vi "DHE_DO_IMREAD_CONT.vi"(8 "error in":errorcluster) -> (0 "error out":errorcluster, 2 "response":string="END READ CONT")   [LabVIEW 2016]
uses:
  Common/public/vis/CMN_FVAR_action.ctl
  SDSU_GBLVariables.vi
  DBSHAND/private/vis/DatabaseHand_Element_Get(I32).vi
  DBSHAND/private/vis/DatabaseHand_Element_Get(double).vi
  DBSHAND/private/vis/DatabaseHand_Element_Set(bool).vi
  c/lib/libarcDHE.so
panel:
  out "remaining elements":string[](array[string])
  out "read prog":i32
  in  "stop":bool
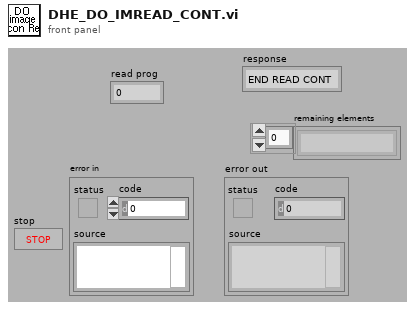
[diagram p1: front panel]
types:
  T1 = typedef "DatabaseHand_RefNum.ctl" = refnum<vi>
  T2 = typedef "CMN_FVAR_action.ctl" = enum16{"read", "write"}
  T3 = enum16{"Idle", "Exposing", "Paused", "AbortExp", "Reading", "AbortRead", "FinishedReading", "Resetting", "Reducing"}
  T4 = typedef "CMN_Buffers.ctl" = cluster{"TotalPixels":u32, "Total image bytes":u32, "Total Phys Buffers":u32, "virtual buf pixels":u32, "virtual bytes size":u32, "Remaining piece":u32, "Transfer_Buf_size":u32}
  T5 = typedef "CMN_ContStatus.ctl" = cluster{"Response":string, "power":bool, "shutter":bool, "artifdata":bool, "idlemode":bool, "reset":bool, "gain":u8, "speed":u8, "resetPCI":bool, "autoshutter":bool, "TempSetPoint":i32, "multipleextensions":bool, "displayImage":bool, "coadding":bool, "images being coadded":i32, "Operation Mode":enum16{"normal", "coadd", "fawler"}, "frames to write":cluster{"subs":bool, "reset":bool, "exposed":bool}, "fawler samples":i32, "write auto":bool, "datatype":string, "frames to display":cluster{"subs":bool, "reset":bool, "exposed":bool}, "sur":i32, "autoclear":bool}
  T6 = enum16{"Idle", "Exposing", "Paused", "AbortExp", "Reading", "AbortRead", "FinishedReading", "Resetting", "Reducing", "Initializing"}
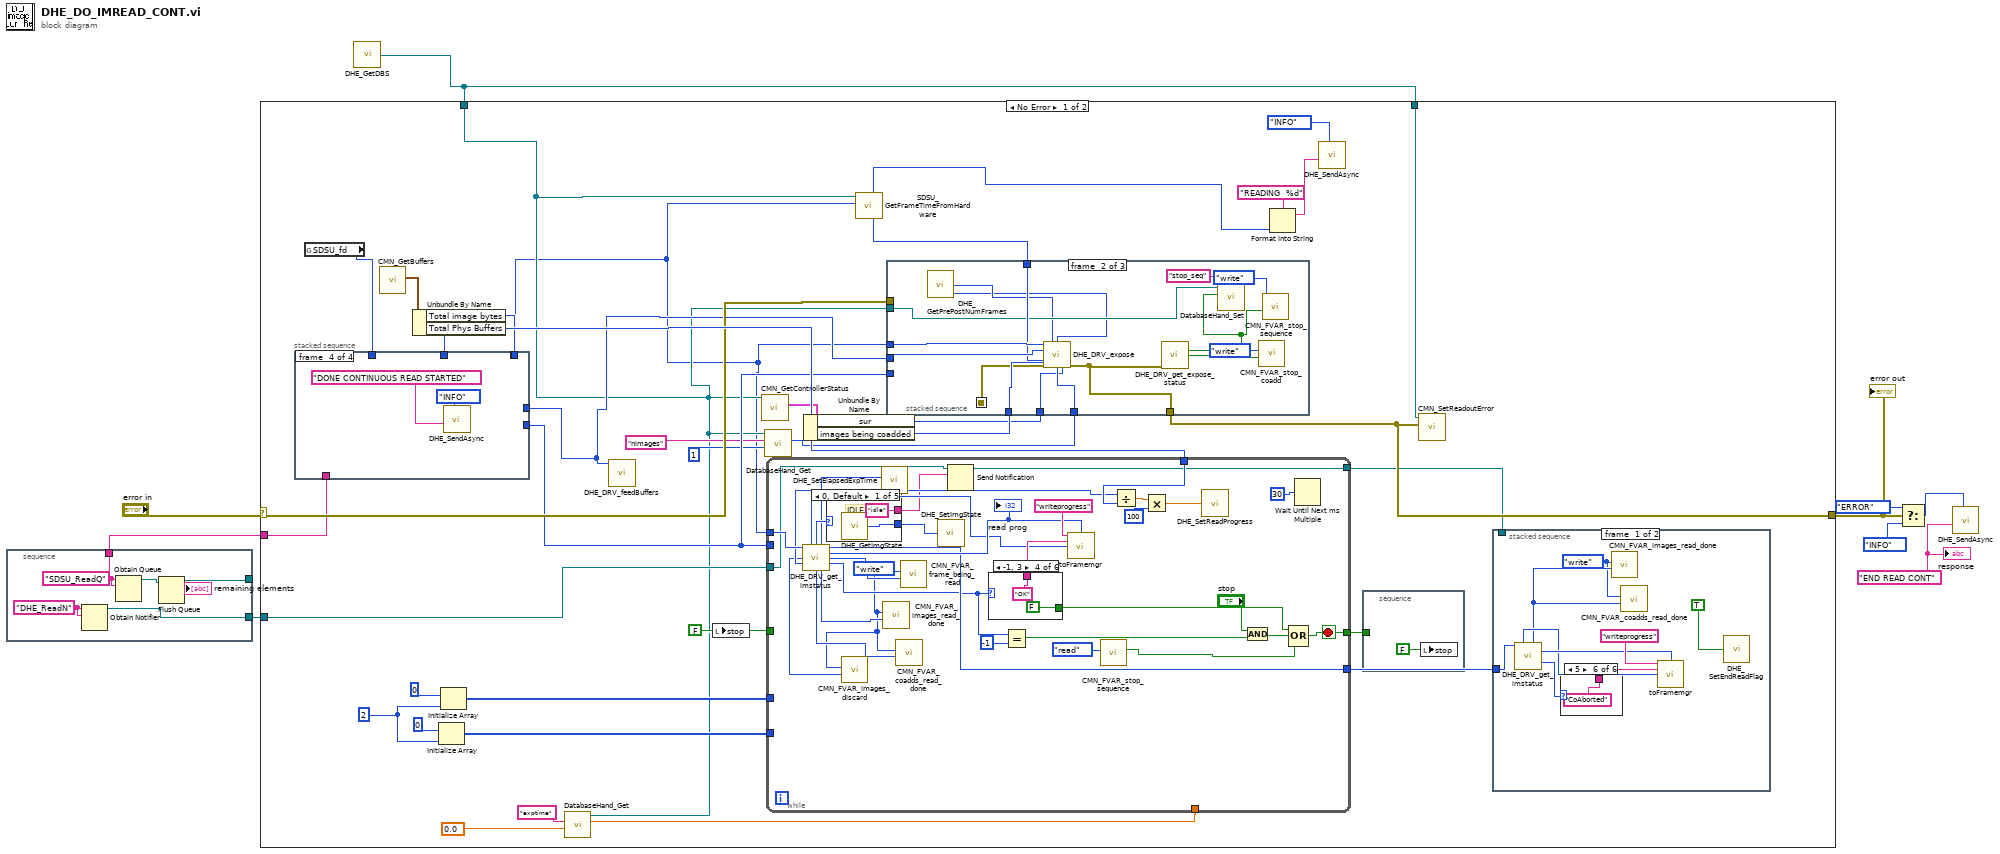
[diagram p0: block diagram]
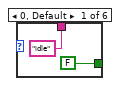
[diagram p2: hidden frame]
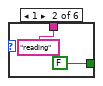
[diagram p3: hidden frame]
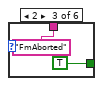
[diagram p4: hidden frame]
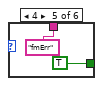
[diagram p5: hidden frame]
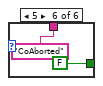
[diagram p6: hidden frame]
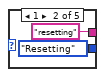
[diagram p7: hidden frame]
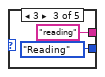
[diagram p8: hidden frame]
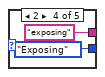
[diagram p9: hidden frame]
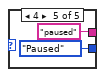
[diagram p10: hidden frame]
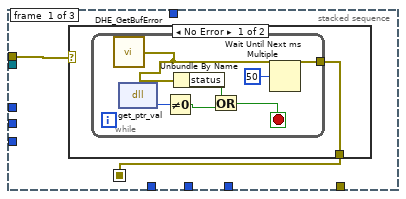
[diagram p11: hidden frame]
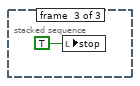
[diagram p13: hidden frame]
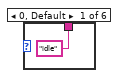
[diagram p14: hidden frame]
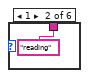
[diagram p15: hidden frame]
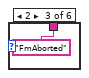
[diagram p16: hidden frame]
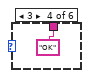
[diagram p17: hidden frame]
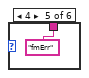
[diagram p18: hidden frame]
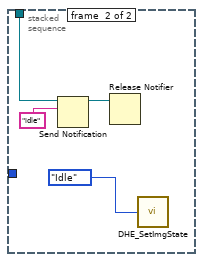
[diagram p19: hidden frame]
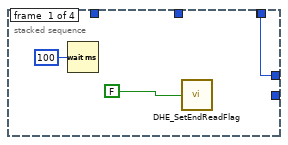
[diagram p20: hidden frame]
diagram:
  w1 = "END READ CONT" ("Message")
  n1 = stacked-sequence {
    tunnel: [w15] -> w8
    tunnel: [w13] -> _
    tunnel: [w10] -> w7
    frame #0 {
      w11 = "DHE_ReadN" ("name (unnamed)")
      w15 = "SDSU_ReadQ" ("name (unnamed)")
      n2 = Obtain Notifier(name (unnamed)=w11, notification data type=w11) -> (notifier out=w10:refnum<notifier>)  [unwired: 2 in, 2 out]
      n3 = Obtain Queue(name (unnamed)=w15, element data type=w15) -> (queue out=w14:refnum<queue>)  [unwired: 3 in, 2 out]
      n4 = Flush Queue(queue=w14) -> (queue out=w13:refnum<queue>, remaining elements=→"remaining elements":string[])  [unwired: 1 in, 1 out]
    }
  }
  n5 = call "DHE_GetDBS.vi"() -> ("DHE_DBSRef"=w6:T1)  [unwired: 9 out]
  n6 = case shown="No Error" "error in" {
    selector: "error in" -> [w43 w169]
    tunnel: [w40 w169] -> w5
    tunnel: w6 -> [w39 _]
    tunnel: w6 -> [w18 _]
    tunnel: w8 -> [w33 _]
    tunnel: w7 -> [w29 _]
    frame No Error {
      w21 = 2 ("dimension size")
      w42 = FALSE ("stop")
      n7 = global read "SDSU_GBLVariables.vi" "SDSU_fd"() -> (w17:i32)
      n8 = call "CMN_GetBuffers.vi"() -> ("BuffersDimensions"=w34:T4)  [unwired: 2 in, 9 out]
      n9 = Unbundle By Name(w34) -> ("Total image bytes"=w31:u32, "Total Phys Buffers"=w51:u32)
      n10 = stacked-sequence {
        tunnel: [_ w157 _ _] -> w41
        tunnel: w51 -> [_ w159 _ _]
        tunnel: w17 -> [_ w158 _ _]
        tunnel: w33 -> [_ _ w161 _]
        tunnel: [w154 _ _ _] -> w30
        tunnel: w31 -> [w154 _ _ _]
        tunnel: [_ w156 _ _] -> w16
        frame #0 {
          n11 = Wait (ms)(milliseconds to wait=u32 100) -> ()  [unwired: 1 out]
          n12 = call "DHE_SetEndReadFlag.vi"("DHE_read_ended"=FALSE ("readout ended")) -> ()  [unwired: 9 out]
        }
        frame #1 {
          n13 = dll-call lib="home/simager/panview/PAN/Modules/SDSU/private/c/lib/libarcDHE.so" fn="clear_exp_vals"() -> ()  [unwired: 3 in, 3 out]
          n14 = call "DHE_DRV_clear_progress_buf.vi"("fd"=w158) -> ("fd"=w156:i32)  [unwired: 1 in, 13 out]
          n15 = dll-call lib="home/simager/panview/PAN/Modules/SDSU/private/c/lib/libarcDHE.so" fn="clear_counters"() -> ()  [unwired: 3 in, 3 out]
          n16 = dll-call lib="home/simager/panview/PAN/Modules/SDSU/private/c/lib/libarcDHE.so" fn="set_bufs_per_frame" label="bufs_per_frame"("total_bufs"=w159) -> ("total_bufs"=w157:i32)  [unwired: 3 in, 3 out]
          n17 = dll-call lib="home/simager/panview/PAN/Modules/SDSU/private/c/lib/libarcDHE.so" fn="clear_discards"() -> ()  [unwired: 3 in, 3 out]
        }
        frame #2 {
          n18 = dll-call lib="home/simager/panview/PAN/Modules/SDSU/private/c/lib/libarcDHE.so" fn="set_status_expo"() -> ()  [unwired: 3 in, 3 out]
          n19 = Concatenate Strings("reading" ("command"), " " ("string"), w161) -> (w160:string)
          n20 = call "CMN_toLogical.vi"("command"=w160) -> ()  [unwired: 10 out]
        }
        frame #3 {
          n21 = call "DHE_SendAsync.vi"("type"=enum16{"ERROR", "WARNING", "INFO", "CHANGED"}."INFO", "Message"="DONE CONTINUOUS READ STARTED") -> ()  [unwired: 10 out]
        }
      }
      n22 = Initialize Array(i16 0, w21) -> (w49:i16[])
      n23 = Initialize Array(0, w21) -> (w50:i32[])
      n24 = call-poly "DatabaseHand_Get.vi"("default value"=0.0, "name"="exptime", "Database RefNum in"=w18) -> ("value"=w32:dbl)  [unwired: 2 in, 6 out]
      n25 = call "DHE_DRV_feedBuffers.vi"("bufsize"=w30) -> ()  [unwired: 10 out]
      n26 = local write "stop"(w42) -> ()
      n27 = call "CMN_GetControllerStatus.vi"("DBS Ref"=w18) -> ("ControllerStatus"=w38:T5)  [unwired: 10 out]
      n28 = call-poly "DatabaseHand_Get.vi"("default value"=1, "name"="nimages", "Database RefNum in"=w18) -> ("value"=w22:i32)  [unwired: 2 in, 6 out]
      n29 = while {
        tunnel: w49 -> [_]
        tunnel: w50 -> [_]
        tunnel: [w73] -> w44
        tunnel: [w70] -> w46
        tunnel: w51 -> [w77]
        tunnel: w16 -> [w79]
        tunnel: w42 -> [_]
        tunnel: w41 -> [_]
        tunnel: w32 -> [_]
        tunnel: w29 -> [w64]
        tunnel: [w63] -> w28
        stop <- w70 stop-if-true
        w55 = CMN_FVAR_action."write" ("action")
        n30 = call "DHE_DRV_get_imstatus.vi"("fd"=w79) -> ("ptr to buffer"=w74:u64, "image status"=w78:i16, "exposure progress"=w60:i32, "fd"=w73:i32, "buff read"=w75:i32, "fowlers_discarded"=w56:i32, "frames read"=w59:i32, "actual_buf_reads"=w72:i32, "frame status"=w68:i32, "coadds done"=w57:i32, "images done"=w58:i32)  [unwired: 1 in, 3 out]
        "read prog" <- w75
        n31 = case shown="0, Default" w78 {
          tunnel: [w96 T3."Resetting" ("ImgState") T3."Reading" ("ImgState") T3."Exposing" ("ImgState") T3."Paused" ("ImgState")] -> w61
          tunnel: ["idle" "resetting" "reading" "exposing" "paused"] -> w62
          frame 0, Default {
            # "IDLE"
            n32 = call "DHE_GetImgState.vi"() -> ("DHE_ImgState"=w96:T6)  [unwired: 9 out]
          }
          frame 1 {
          }
          frame 3 {
          }
          frame 2 {
          }
          frame 4 {
          }
        }
        n33 = call "CMN_FVAR_images_discard.vi"("value in"=w56, "action"=w55) -> ()  [unwired: 9 out]
        n34 = call "DHE_SetElapsedExpTime.vi"("ElapsedExpTime"=w60) -> ()  [unwired: 11 out]
        n35 = call "CMN_FVAR_images_read_done.vi"("value in"=w58, "action"=w55) -> ()  [unwired: 9 out]
        n36 = call "CMN_FVAR_coadds_read_done.vi"("value in"=w57, "action"=w55) -> ()  [unwired: 9 out]
        n37 = call "CMN_FVAR_frame_being_read.vi"("value in"=w59, "action"=w55) -> ()  [unwired: 9 out]
        n38 = call "DHE_SetImgState.vi"("DHE_ImgState"=w61) -> ()  [unwired: 9 out]
        n39 = Send Notification(notification=w62, notifier=w64) -> (notifier out=w63:refnum<notifier>)  [unwired: 1 in, 1 out]
        n40 = case shown="-1, 3" w68 {
          tunnel: ["idle" "reading" "FmAborted" "OK" "fmErr" "CoAborted"] -> w76
          tunnel: [FALSE FALSE TRUE FALSE TRUE FALSE] -> w65
          frame 0, Default {
          }
          frame 1 {
          }
          frame 2 {
          }
          frame -1, 3 {
          }
          frame 4 {
          }
          frame 5 {
          }
        }
        n41 = Equal?(x=w68, y=-1) -> (x = y?=w66:bool)
        n42 = call "toFramemgr.vi"("command"="writeprogress", "progress"=w75, "arg"=w76, "bufpointer"=w74) -> ()  [unwired: 5 in, 7 out]
        n43 = call "CMN_FVAR_stop_sequence.vi"("action"=CMN_FVAR_action."read") -> ("value out"=w52:bool)  [unwired: 1 in, 8 out]
        n44 = Divide(x=w72, y=w77) -> (x/y=w81:dbl)
        n45 = Multiply(x=w81, y=100) -> (x*y=w54:dbl)
        n46 = call "DHE_SetReadProgress.vi"("ReadProgress"=w54) -> ()  [unwired: 11 out]
        n47 = And(x="stop", y=w66) -> (x .and. y?=w69:bool)
        n48 = Compound Arithmetic op=OR(w65, w69, w52) -> (w70:bool)
        n49 = Wait Until Next ms Multiple(millisecond multiple=u32 30) -> ()  [unwired: 1 out]
      }
      n50 = Unbundle By Name(w38) -> ("sur"=w37:i32, "images being coadded"=w45:i32)
      n51 = call "SDSU_GetFrameTimeFromHardware.vi"("fd"=w16, "Database Ref"=w18) -> ("idle time"=w20:u32, "total exp time"=w19:u32)  [unwired: 1 in, 7 out]
      n52 = stacked-sequence {
        seq-local: [w108 _ _] -> [_ w128 _]
        tunnel: w30 -> [_ w131 _]
        tunnel: w16 -> [_ w132 _]
        tunnel: [_ w126 _] -> w40
        tunnel: w43 -> [w107 _ _]
        tunnel: w22 -> [_ w130 _]
        tunnel: w45 -> [_ w129 _]
        tunnel: w20 -> [_ w127 _]
        tunnel: w41 -> [_ _ _]
        tunnel: w37 -> [_ w125 _]
        tunnel: w18 -> [_ w124 _]
        frame #0 {
          n53 = case shown="No Error" w107 {
            selector: w107 -> [_ w116]
            tunnel: [w109 w116] -> w108
            frame No Error {
              n54 = while {
                tunnel: [w110] -> w109
                stop <- w112 stop-if-true
                n55 = call "DHE_GetBufError.vi"() -> ("DHE_BufError"=w110:errorcluster)  [unwired: 9 out]
                n56 = dll-call lib="home/simager/panview/PAN/Modules/SDSU/private/c/lib/libarcDHE.so" fn="get_ptr_val"() -> (w115:u32)  [unwired: 3 in, 2 out]
                n57 = Not Equal To 0?(x=w115) -> (x != 0?=w114:bool)
                n58 = Unbundle By Name(w110) -> ("status"=w111:bool)
                n59 = Or(x=w111, y=w114) -> (x .or. y?=w112:bool)
                n60 = Wait Until Next ms Multiple(millisecond multiple=u32 50) -> ()  [unwired: 1 out]
              }
            }
            frame Error {
            }
          }
        }
        frame #1 {
          n61 = call "DHE_GetPrePostNumFrames.vi"() -> ("DHE_PreExpose"=w122:i32, "DHE_PostExpose"=w121:i32)  [unwired: 8 out]
          n62 = call "DHE_DRV_expose.vi"("fd"=w132, "num_prevex"=w122, "num_postex"=w121, "bytes_to_receive"=w131, "expt_time"=w127, "error in (no error)"=w128, "num_coadds"=w129, "npics"=w130, "num_sur"=w125) -> ("error out"=w126:errorcluster)  [unwired: 1 in, 5 out]
          n63 = call "DHE_DRV_get_expose_status.vi"("error in (no error)"=w126) -> ("sequence stoped"=w120:bool, "coadd stoped"=w118:bool)  [unwired: 13 out]
          n64 = call-poly "DatabaseHand_Set.vi"("name"="stop_seq", "value"=w120, "Database RefNum in"=w124) -> ()  [unwired: 5 in, 4 out]
          n65 = call "CMN_FVAR_stop_coadd.vi"("value in"=w118, "action"=CMN_FVAR_action."write") -> ()  [unwired: 9 out]
          n66 = call "CMN_FVAR_stop_sequence.vi"("value in"=w120, "action"=CMN_FVAR_action."write") -> ()  [unwired: 9 out]
        }
        frame #2 {
          n67 = local write "stop"(TRUE ("stop")) -> ()
        }
      }
      n68 = Format Into String(format string="READING  %d", w19) -> (resulting string=w25:string)  [unwired: 2 in, 1 out]
      n69 = call "DHE_SendAsync.vi"("type"=enum16{"ERROR", "WARNING", "INFO", "CHANGED"}."INFO", "Message"=w25) -> ()  [unwired: 2 in, 8 out]
      n70 = stacked-sequence {
        tunnel: w46 -> [_]
        frame #0 {
          n71 = local write "stop"(FALSE ("stop")) -> ()
        }
      }
      n72 = call "CMN_SetReadoutError.vi"("readout error"=w40, "Database RefNum in"=w39) -> ()  [unwired: 1 in, 9 out]
      n73 = stacked-sequence {
        tunnel: w44 -> [w141 _]
        tunnel: w28 -> [_ w152]
        frame #0 {
          w134 = CMN_FVAR_action."write" ("action")
          n74 = call "DHE_DRV_get_imstatus.vi"("fd"=w141) -> ("ptr to buffer"=w137:u64, "buff read"=w138:i32, "frame status"=w140:i32, "images done"=w135:i32)  [unwired: 1 in, 10 out]
          n75 = case shown="5" w140 {
            tunnel: ["idle" "reading" "FmAborted" "OK" "fmErr" "CoAborted"] -> w139
            frame 0, Default {
            }
            frame 1 {
            }
            frame 2 {
            }
            frame 3 {
            }
            frame 4 {
            }
            frame 5 {
            }
          }
          n76 = call "CMN_FVAR_images_read_done.vi"("value in"=w135, "action"=w134) -> ()  [unwired: 9 out]
          n77 = call "CMN_FVAR_coadds_read_done.vi"("value in"=w135, "action"=w134) -> ()  [unwired: 9 out]
          n78 = call "toFramemgr.vi"("command"="writeprogress", "progress"=w138, "arg"=w139, "bufpointer"=w137) -> ()  [unwired: 5 in, 7 out]
          n79 = call "DHE_SetEndReadFlag.vi"("DHE_read_ended"=TRUE ("readout ended")) -> ()  [unwired: 9 out]
        }
        frame #1 {
          n80 = Send Notification(notification="idle", notifier=w152) -> (notifier out=w151:refnum<notifier>)  [unwired: 1 in, 1 out]
          n81 = Release Notifier(notifier=w151) -> ()  [unwired: 1 in, 4 out]
          n82 = call "DHE_SetImgState.vi"("DHE_ImgState"=T3."Idle" ("ImgState")) -> ()  [unwired: 9 out]
        }
      }
    }
    frame Error {
      n83 = Unbundle By Name(w169) -> ("source"=w168:string)
      n84 = Concatenate Strings("error " ("command"), w168) -> (w167:string)
      n85 = call "CMN_toLogical.vi"("command"=w167) -> ()  [unwired: 10 out]
      n86 = call "DHE_SetImgState.vi"("DHE_ImgState"=T3."Idle" ("ImgState")) -> ()  [unwired: 9 out]
    }
  }
  "error out" <- w5
  n87 = Select(t=enum16{"ERROR", "WARNING", "INFO", "CHANGED"}."ERROR", s=w5, f=enum16{"ERROR", "WARNING", "INFO", "CHANGED"}."INFO" ("type")) -> (s? t:f=w2:enum16{"ERROR", "WARNING", "INFO", "CHANGED"})
  n88 = call "DHE_SendAsync.vi"("type"=w2, "Message"=w1) -> ()  [unwired: 10 out]
  "response" <- w1
